vi "SetWAFactor.vi"(8 "error in (no error)":errorcluster, 11 "Laser Diode Controller in":refnum<class "KLD101.lvclass">) -> (0 "error out":errorcluster, 3 "Laser Diode Controller out":refnum<class "KLD101.lvclass">)   [LabVIEW 2016, in "Laser Diode Controller.lvlib" / "KLD101.lvclass"]
uses:
  KLD101.lvclass
  KLD101.lvclass/KLD101.ctl
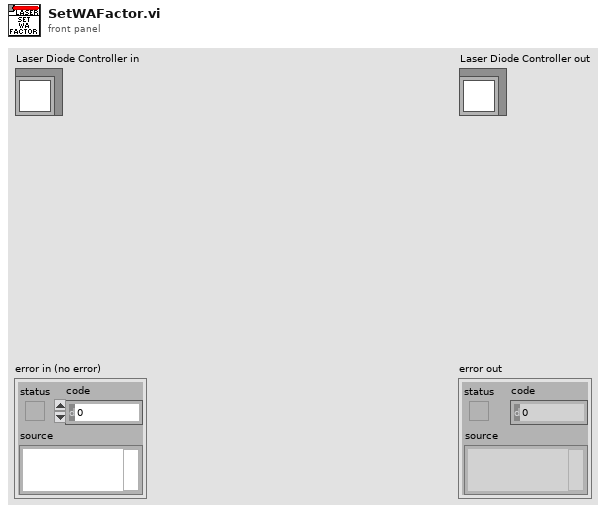
[diagram p1: front panel]
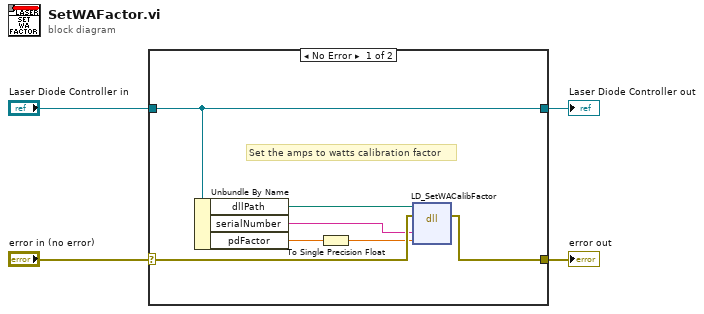
[diagram p0: block diagram]
diagram:
  n1 = case shown="No Error" "error in (no error)" {
    selector: "error in (no error)" -> [w10 w13]
    tunnel: [w9 w13] -> w3
    tunnel: [w11 w12] -> w1
    tunnel: "Laser Diode Controller in" -> [w11 w12]
    frame No Error {
      # "Set the amps to watts calibration factor"
      n2 = Unbundle By Name(w11) -> ("dllPath"=w5:path, "serialNumber"=w8:string, "pdFactor"=w7:sgl)
      n3 = To Single Precision Float(number=w7) -> (single precision float=w6:sgl)
      n4 = dll-call lib="C:/IDEXX Software/Collimation/data/Thorlabs.MotionControl.KCube.LaserDiode.dll" fn="LD_SetWACalibFactor"(path in=w5, error in=w10, "serialNumber"=w8, "calibFactor"=w6) -> (error out=w9:errorcluster)  [unwired: 4 in, 1 out]
    }
    frame Error {
    }
  }
  "error out" <- w3
  "Laser Diode Controller out" <- w1
